vi "onTestDiscovery.vi"(8 "error in (no error)":errorcluster, 11 "Test Runner.Folder in":refnum<class "Test Runner.Folder.lvclass">) -> (0 "error out":errorcluster, 2 "Tests VIs":path[](array[path]), 3 "Test Runner.Folder out":refnum<class "Test Runner.Folder.lvclass">)   [LabVIEW 2013, in "Caraya.lvlib" / "Test Runner.Folder.lvclass"]
uses:
  Test Runner.Folder.lvclass
  Test Runner.Folder.lvclass/Test Runner.Folder.ctl
  <userlib>/_OpenG.lib/file/file.llb/File Exists - Scalar__ogtk.vi
  <userlib>/_OpenG.lib/file/file.llb/Valid Path - Traditional__ogtk.vi
  Test/Define Test.vi
  <userlib>/_OpenG.lib/file/file.llb/Build Path - File Names Array__ogtk.vi
  Test/Test.lvclass
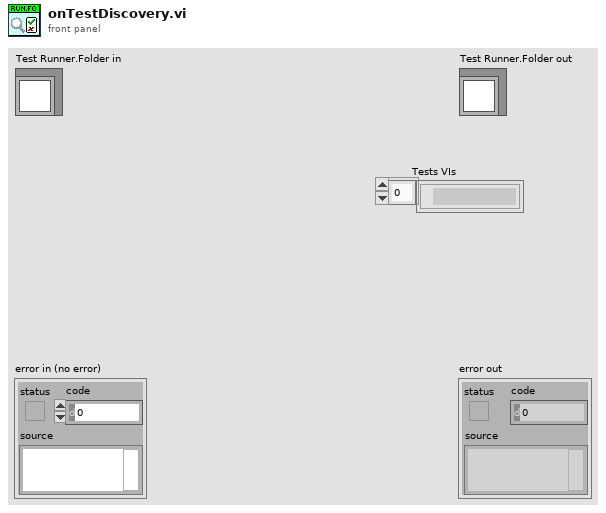
[diagram p1: front panel]
types:
  T1 = typedef "NI_FileType.lvlib/LVFileType.ctl" = enum32{"Invalid file", "Unknown type", "Instrument", "Control", "Polymorphic VI", "Project", "Library", "LVClass", "XControl", "XNode", "Shared library", ".NET assembly", "ActiveX interface", "CIN", "Run-time menu", "Palette menu", "Help file", "LLB", "XNode Edit Dependency", "Class Private Data Control", "Statechart", "MathScript .m file", "Ladder Diagram", "LVLibp"}
  T2 = cluster{"path":path, "delimited name":string, "type":T1, "iState":u32, "iStyle":u16, "wStyle":u16, "buttons":u16, "viflags":u32, "viflags2":u32, "links":u32[]}[]
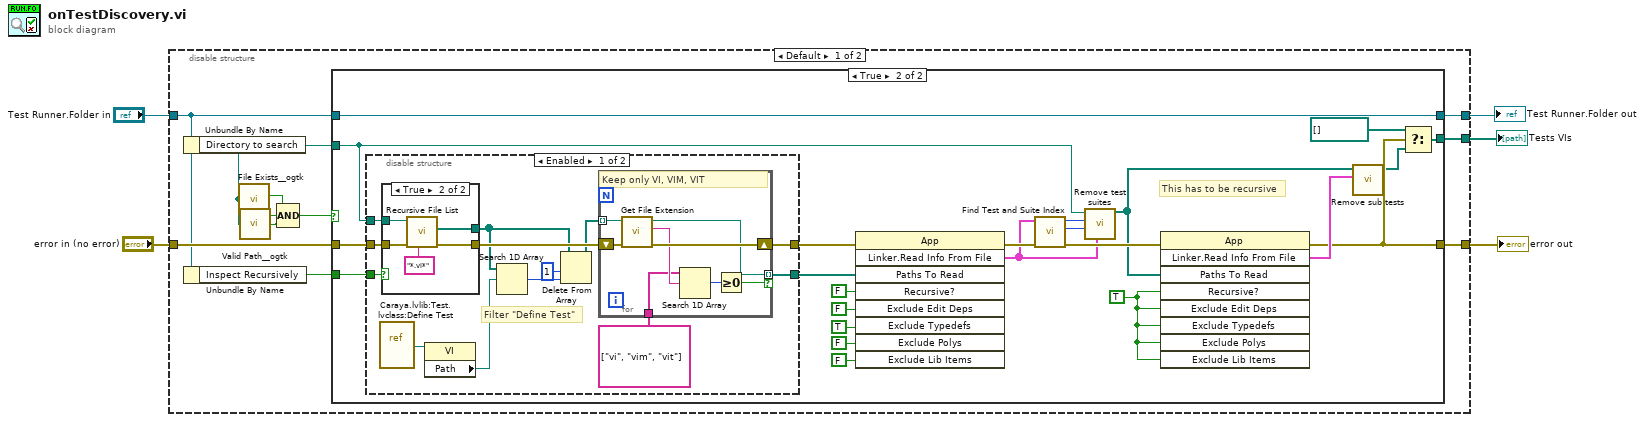
[diagram p0: block diagram]
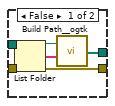
[diagram p3: hidden frame]
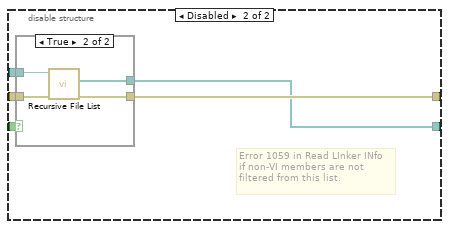
[diagram p4: hidden frame]
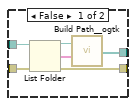
[diagram p5: hidden frame]
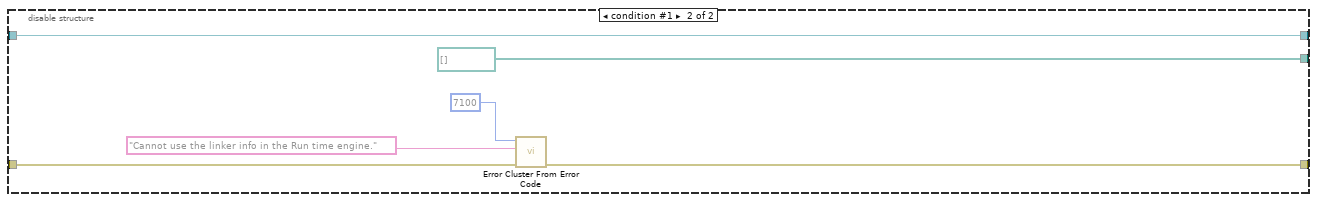
[diagram p6: hidden frame]
diagram:
  n1 = disable-structure shown="Default" {
    disable-tunnel: [w11 w90] -> w2
    disable-tunnel: "Test Runner.Folder in" -> [w7 w89]
    disable-tunnel: [w10 w89] -> w4
    disable-tunnel: [w9 path[] [] ("Test VIs")] -> w3
    disable-tunnel: "error in (no error)" -> [w8 w87]
    frame condition #0 (active) {
      n2 = Unbundle By Name(w7) -> ("Directory to search"=w14:path)
      n3 = Unbundle By Name(w7) -> ("Inspect Recursively"=w6:bool)
      n4 = call-poly <userlib>:"File Exists__ogtk.vi"("file path"=w14) -> ("is directory"=w13:bool, "exists"=w15:bool)  [unwired: 6 in]
      n5 = call-poly <userlib>:"Valid Path__ogtk.vi"("path"=w14) -> ("valid"=w16:bool)
      n6 = Compound Arithmetic op=AND(w13, w15, w16) -> (w12:bool)
      n7 = case shown="True" w12 {
        tunnel: w6 -> [_ w30]
        tunnel: [w17 w29] -> w11
        tunnel: [_ w27] -> w9
        tunnel: w14 -> [_ w21]
        tunnel: w7 -> [w18 w25]
        tunnel: [w18 w25] -> w10
        tunnel: w8 -> [w17 w19]
        frame False {
        }
        frame True {
          w32 = TRUE ("Recursive?")
          # "This has to be recursive"
          n8 = disable-structure shown="Enabled" {
            disable-tunnel: w30 -> [w54 w76]
            disable-tunnel: [w52 w74] -> w24
            disable-tunnel: [w51 w73] -> w23
            disable-tunnel: w21 -> [w50 w75]
            disable-tunnel: w19 -> [w42 _]
            frame Enabled {
              # "Filter \"Define Test\""
              n9 = vi-ref "Caraya.lvlib:Test.lvclass:Define Test.vi"() -> (w48:refnum<vi>)
              n10 = case shown="True" w54 {
                tunnel: [w63 w72] -> w43
                tunnel: [w66 w71] -> w53
                tunnel: w50 -> [w67 w70]
                tunnel: w42 -> [_ w68]
                frame False {
                  n11 = List Folder(path=w67) -> (path out=w65:path, filenames=w64:string[], error out=w66:errorcluster)  [unwired: 3 in, 1 out]
                  n12 = call-poly <userlib>:"Build Path__ogtk.vi"("name or relative path"=w64, "base path"=w65) -> ("appended path"=w63:path[])
                }
                frame True {
                  n13 = call <vilib>:"Recursive File List.vi"("pattern"="*.vi*", "error in (no error)"=w68, "Folder Path"=w70) -> ("error out"=w71:errorcluster, "All Files in Dir"=w72:path[])  [unwired: 4 in, 3 out]
                }
              }
              n14 = property class="VI"(reference=w48) -> ("Path"=w47:path)  [unwired: 1 in, 2 out]
              n15 = Search 1D Array(1D array=w43, element=w47) -> (index of element=w45:i32)  [unwired: 1 in]
              n16 = Delete From Array(array=w43, length=1, index=w45) -> (array with subset deleted=w46:path[])  [unwired: 1 out]
              n17 = for {
                tunnel: w46 -> [w62] mode=indexing
                shift-right: [w60] -> w52
                shift-left: w53 -> [w61]
                tunnel: [w59] -> w51 mode=indexing if=w55
                tunnel: string[] ["vi", "vim", "vit"] -> [w57]
                # "Keep only VI, VIM, VIT"
                n18 = call <vilib>:"Get File Extension.vi"("error in (no error)"=w61, "file"=w62) -> ("error out"=w60:errorcluster, "lowercase file extension"=w58:string, "dup file"=w59:path)  [unwired: 6 in, 1 out]
                n19 = Search 1D Array(1D array=w57, element=w58) -> (index of element=w56:i32)  [unwired: 1 in]
                n20 = Greater Or Equal To 0?(x=w56) -> (x >= 0?=w55:bool)
              }
            }
            frame Disabled {
              # "Error 1059 in Read LInker INfo\nif non-VI members are not\nfiltered from this list."
              n21 = case shown="True" w76 {
                tunnel: _ -> [w81 w86]
                tunnel: [w77 w85] -> w73
                tunnel: [w80 w84] -> w74
                tunnel: w75 -> [w82 w83]
                frame False {
                  n22 = List Folder(path=w82, error in=w81) -> (path out=w79:path, filenames=w78:string[], error out=w80:errorcluster)  [unwired: 2 in, 1 out]
                  n23 = call-poly <userlib>:"Build Path__ogtk.vi"("name or relative path"=w78, "base path"=w79) -> ("appended path"=w77:path[])
                }
                frame True {
                  n24 = call <vilib>:"Recursive File List.vi"("error in (no error)"=w86, "Folder Path"=w83) -> ("error out"=w84:errorcluster, "All Files in Dir"=w85:path[])  [unwired: 5 in, 3 out]
                }
              }
            }
          }
          n25 = invoke class="App" method="Linker.Read Info From File"(error in=w24, "Paths To Read"=w23, "Recursive?"=FALSE, "Exclude Edit Deps"=FALSE ("Exclude Edit Time Dependencies"), "Exclude Typedefs"=TRUE, "Exclude Polys"=FALSE ("Exclude Poly VIs"), "Exclude Lib Items"=FALSE ("Exclude Unused Library Items")) -> (error out=w36:errorcluster, "Linker.Read Info From File"=w22:T2)  [unwired: 2 in, 7 out]
          n26 = call "Find Test and Suite Index.vi"("error in (no error)"=w36, "Linker.Read Info From File"=w22) -> ("error out"=w33:errorcluster, "Define Test index"=w34:i32, "Define Test Suite index"=w35:i32)  [unwired: 7 in]
          n27 = call "Remove test suites.vi"("Linker.Read Info From File"=w22, "Define Test index"=w34, "Define Test Suite index"=w35, "Directory to search"=w21) -> ("Tests"=w20:path[])  [unwired: 7 in]
          n28 = invoke class="App" method="Linker.Read Info From File"(error in=w33, "Paths To Read"=w20, "Recursive?"=w32, "Exclude Edit Deps"=w32, "Exclude Typedefs"=w32, "Exclude Polys"=w32, "Exclude Lib Items"=w32) -> (error out=w29:errorcluster, "Linker.Read Info From File"=w31:T2)  [unwired: 2 in, 7 out]
          n29 = call "Remove sub tests.vi"("Linker.Read Info From File"=w31, "Tests"=w20) -> ("Array"=w28:path[])  [unwired: 9 in]
          n30 = Select(t=path[] [], s=w29, f=w28) -> (s? t:f=w27:path[])
        }
      }
    }
    frame condition #1 {
      n31 = call <vilib>:"Error Cluster From Error Code.vi"("error in (no error)"=w87, "error message (\"\")"="Cannot use the linker info in the Run time engine." ("error message (\"\")"), "error code (0)"=7100) -> ("error out"=w90:errorcluster)  [unwired: 6 in]
    }
  }
  "error out" <- w2
  "Test Runner.Folder out" <- w4
  "Tests VIs" <- w3
